vi "Deploy.vi"(11 "target in":refnum<class "Base Target.lvclass">) -> (3 "target out":refnum<class "Base Target.lvclass">)   [LabVIEW 2020, in "NI_TargetHelper.lvlib" / "Base Target.lvclass"]
uses:
  <vilib>/TargetSupport/NI_TargetHelper/Base Target/Base Target.lvclass
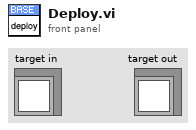
[diagram p1: front panel]
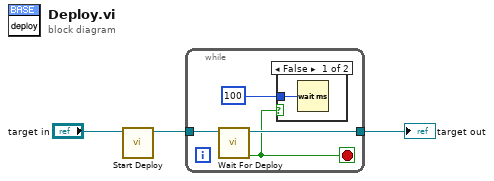
[diagram p0: block diagram]
diagram:
  n1 = call-dynamic "Start Deploy.vi"("target in"="target in") -> ("target out"=w3:refnum<class "Base Target.lvclass">)  [unwired: 10 in]
  n2 = while {
    tunnel: w3 -> [w7]
    tunnel: [w6] -> w1
    stop <- w5 stop-if-true
    n3 = call-dynamic "Wait For Deploy.vi"("target in"=w7) -> ("deployed"=w5:bool, "target out"=w6:refnum<class "Base Target.lvclass">)  [unwired: 9 in]
    n4 = case shown="False" w5 {
      tunnel: u32 100 -> [w8 _]
      frame False {
        n5 = Wait (ms)(milliseconds to wait=w8) -> ()  [unwired: 1 out]
      }
      frame True {
      }
    }
  }
  "target out" <- w1
